vi "WFT I2C Write.vi"(0 "WaveForms Session In":T1, 1 "adr8Bits":u8, 5 "rgbTx":u8[](array[numeric]), 11 "Error In":errorcluster) -> (4 "WaveForms Session Out":T1, 6 "ret":i32, 8 "pNak":i32, 15 "Error Out":errorcluster)   [LabVIEW 2020, in "lv_waveforms_toolkit.lvlib"]
uses:
  lv_waveforms_toolkit.lvlib
  WFT Session.ctl
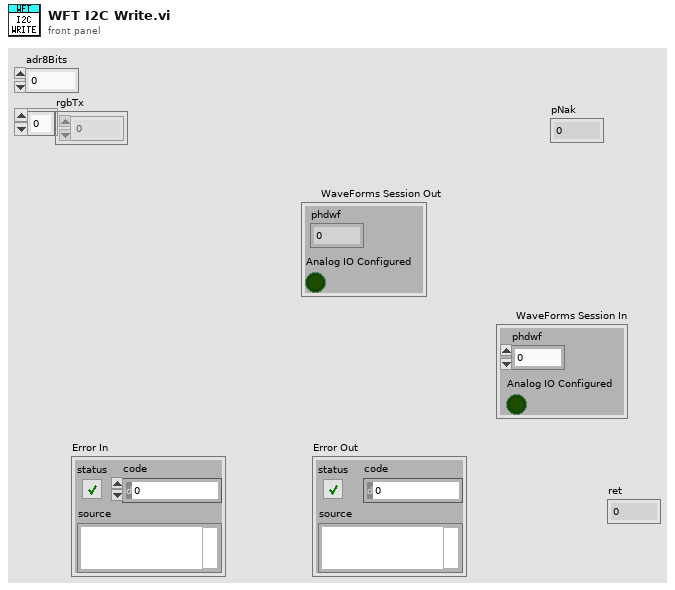
[diagram p1: front panel]
types:
  T1 = typedef "lv_waveforms_toolkit.lvlib/WFT Session.ctl" = cluster{"phdwf":i32, "Analog IO Configured":bool}
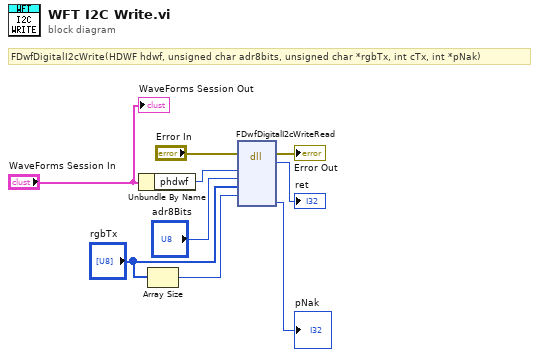
[diagram p0: block diagram]
diagram:
  # "FDwfDigitalI2cWrite(HDWF hdwf, unsigned char adr8bits, unsigned char *rgbTx, int cTx, int *pNak)"
  n1 = Unbundle By Name("WaveForms Session In") -> ("phdwf"=w5:i32)
  n2 = Array Size(array="rgbTx") -> (size(s)=w1:i32)
  n3 = dll-call lib="dwf" fn="FDwfDigitalI2cWriteRead"(error in="Error In", "phdwf"=w5, "adr8Bits"="adr8Bits", "rgbTx"="rgbTx", "cTx"=w1) -> (error out=→"Error Out":errorcluster, "return type"=→"ret":i32, "pNak"=→"pNak":i32)  [unwired: 7 in, 1 out]
  "WaveForms Session Out" <- "WaveForms Session In"
